vi "Sensor Changes.vi"(7 "Index":i32, 9 "New":string, 10 "Old":string, 11 "Sensor DAO Class In":refnum<class "Sensor DAO Class.lvclass">) -> (3 "Sensor DAO Class Out":refnum<class "Sensor DAO Class.lvclass">)   [LabVIEW 2013]
uses:
  \\psf\projects/NSEL OM/XControls/Sensor DAO Class.lvclass
  \\psf\projects/NSEL OM/XControls/Sensor DAO Class.lvclass/Sensor DAO Class.ctl
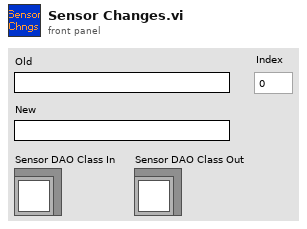
[diagram p1: front panel]
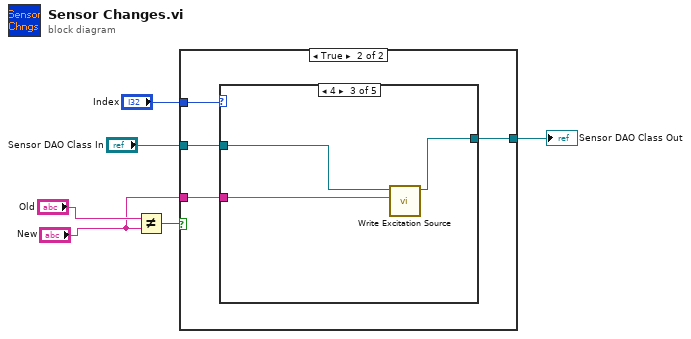
[diagram p0: block diagram]
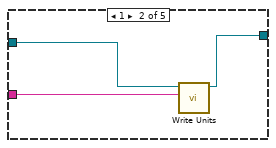
[diagram p4: hidden frame]
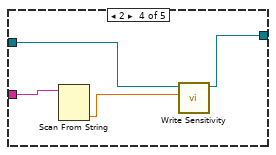
[diagram p5: hidden frame]
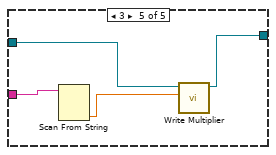
[diagram p6: hidden frame]
diagram:
  n1 = Not Equal?(x="Old", y="New") -> (x != y?=w5:bool)
  n2 = case shown="True" w5 {
    tunnel: "Index" -> [_ w11]
    tunnel: "New" -> [_ w10]
    tunnel: "Sensor DAO Class In" -> [w7 w9]
    tunnel: [w7 w8] -> w1
    frame False {
    }
    frame True {
      n3 = case shown="4" w11 {
        tunnel: w10 -> [_ w15 w18 w22 w26]
        tunnel: w9 -> [w12 w14 w17 w21 w25]
        tunnel: [w12 w13 w16 w20 w24] -> w8
        frame 0, Default {
        }
        frame 1 {
          n4 = call "Write Units.vi"("Units"=w15, "Sensor DAO Class in"=w14) -> ("Sensor DAO Class out"=w13:refnum<class "Sensor DAO Class.lvclass">)  [unwired: 8 in, 1 out]
        }
        frame 4 {
          n5 = call "Write Excitation Source.vi"("Excitation Source"=w18, "Sensor DAO Class in"=w17) -> ("Sensor DAO Class out"=w16:refnum<class "Sensor DAO Class.lvclass">)  [unwired: 8 in, 1 out]
        }
        frame 2 {
          n6 = Scan From String(input string=w22) -> (output 1=w19:dbl)  [unwired: 4 in, 3 out]
          n7 = call "Write Sensitivity.vi"("Sensitivity"=w19, "Sensor DAO Class in"=w21) -> ("Sensor DAO Class out"=w20:refnum<class "Sensor DAO Class.lvclass">)  [unwired: 8 in, 1 out]
        }
        frame 3 {
          n8 = Scan From String(input string=w26) -> (output 1=w23:dbl)  [unwired: 4 in, 3 out]
          n9 = call "Write Multiplier.vi"("Multiplier"=w23, "Sensor DAO Class in"=w25) -> ("Sensor DAO Class out"=w24:refnum<class "Sensor DAO Class.lvclass">)  [unwired: 8 in, 1 out]
        }
      }
    }
  }
  "Sensor DAO Class Out" <- w1
